vi "Periodic Tasks.vi"(0 "error in":errorcluster) -> ()   [LabVIEW 2018]
doc: "This VI runs in parallel to other tasks. It can contain as many user-defined periodic loops as you need. These can carry out PID or other sorts of timed response."
uses:
  dsinstructions.vi
  sensors.vi
  dsdata.vi
  constants.vi
  robotmodes.vi
  refnums.vi
  outputs.vi
panel:
  in  "LED Setting":dbl(slide) min=-1.0 max=1.0 step=0.01 scale=-1.0..1.0
  out "PID Tracking":cluster{"Goal Wheel Position":dbl, dbl}(graph)={"Goal Wheel Position"=0.0, -90.17571233858979}
  out "Contribution Tracking":cluster{dbl, dbl, dbl}(graph)
  in  "Swerve N-Int":i32=10 caption="N-Int"
  in  "Swerve N-Diff":i32=10 caption="N-Diff"
  in  "Swerve Kd":dbl
  in  "Swerve Ki":dbl
  in  "Swerve Kp":dbl=0.005
  out "Drive Sequencer":i32
  out "Subsystem Action":path
  out "Time Since Latch (ms)":u32
  out "Subsystem Sequencer":i32
  out "Drive Action":string
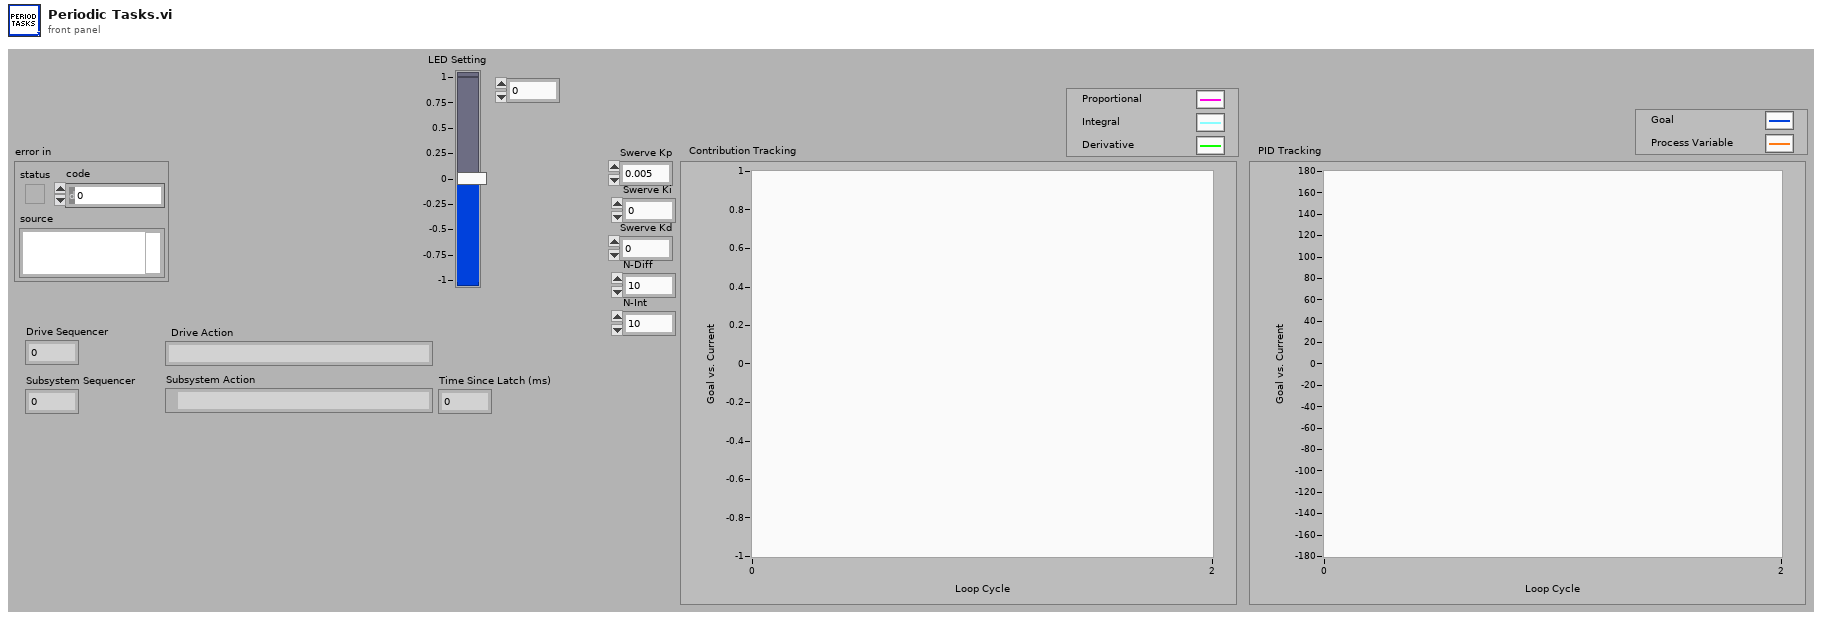
[diagram p1: front panel]
types:
  T1 = typedef "WPI_MotorControlDeviceRef.ctl" = cluster{"DeviceStatus":errorcluster, "Type":T2, "PWM":cluster{"PWM Channel":T3, "DeadBand":T4}, "CAN":cluster{"Device Number":u8, "SetOutput VI Ref":variant, "GetOutput VI Ref":variant, "Enable VI Ref":variant, "Disable VI Ref":variant, "Data":variant}, "Invert":bool, "DIO PWM":cluster{"PWM \"Enable\" Channel":T3, "DIOChannel":T5, "PWM Rate":dbl}}
  T2 = typedef "WPI_MotorControlType.ctl" = enum16{"PWM", "CAN", "DIO PWM"}
  T3 = typedef "FPGA_DIOPWMChannel.ctl" = enum8{"PWM 0", "PWM 1", "PWM 2", "PWM 3", "PWM 4", "PWM 5", "PWM 6", "PWM 7", "PWM 8", "PWM 9", "PWM MXP 0", "PWM MXP 1", "PWM MXP 2", "PWM MXP 3", "PWM MXP 4", "PWM MXP 5", "PWM MXP 6", "PWM MXP 7", "PWM MXP 8", "PWM MXP 9", "Invalid"}
  T4 = typedef "WPI_PWMDeadband.ctl" = cluster{"Name":string, "maxPositivePwm":i32, "minPositivePwm":i32, "centerPwm":i32, "maxNegativePwm":i32, "minNegativePwm":i32, "angularRange":u16}
  T5 = typedef "FPGA_DIOChannel.ctl" = enum8{"DIO 0", "DIO 1", "DIO 2", "DIO 3", "DIO 4", "DIO 5", "DIO 6", "DIO 7", "DIO 8", "DIO 9", "DIO MXP 0", "DIO MXP 1", "DIO MXP 2", "DIO MXP 3", "DIO MXP 4", "DIO MXP 5", "DIO MXP 6", "DIO MXP 7", "DIO MXP 8", "DIO MXP 9", "DIO MXP 10", "DIO MXP 11", "DIO MXP 12", "DIO MXP 13", "DIO MXP 14", "DIO MXP 15", "SPI Port CS1", "SPI Port CS2", "SPI Port CS3", "SPI Port MISO", "SPI Port MOSI", "Invalid"}
  T6 = typedef "WPI_DriverStationRobotMode2.ctl" = enum16{"Autonomous Disabled", "Autonomous Enabled", "Teleop Disabled", "Teleop Enabled", "Disconnected", "Finish", "Test Disabled", "Test Enabled", "Emergency Stopped"}
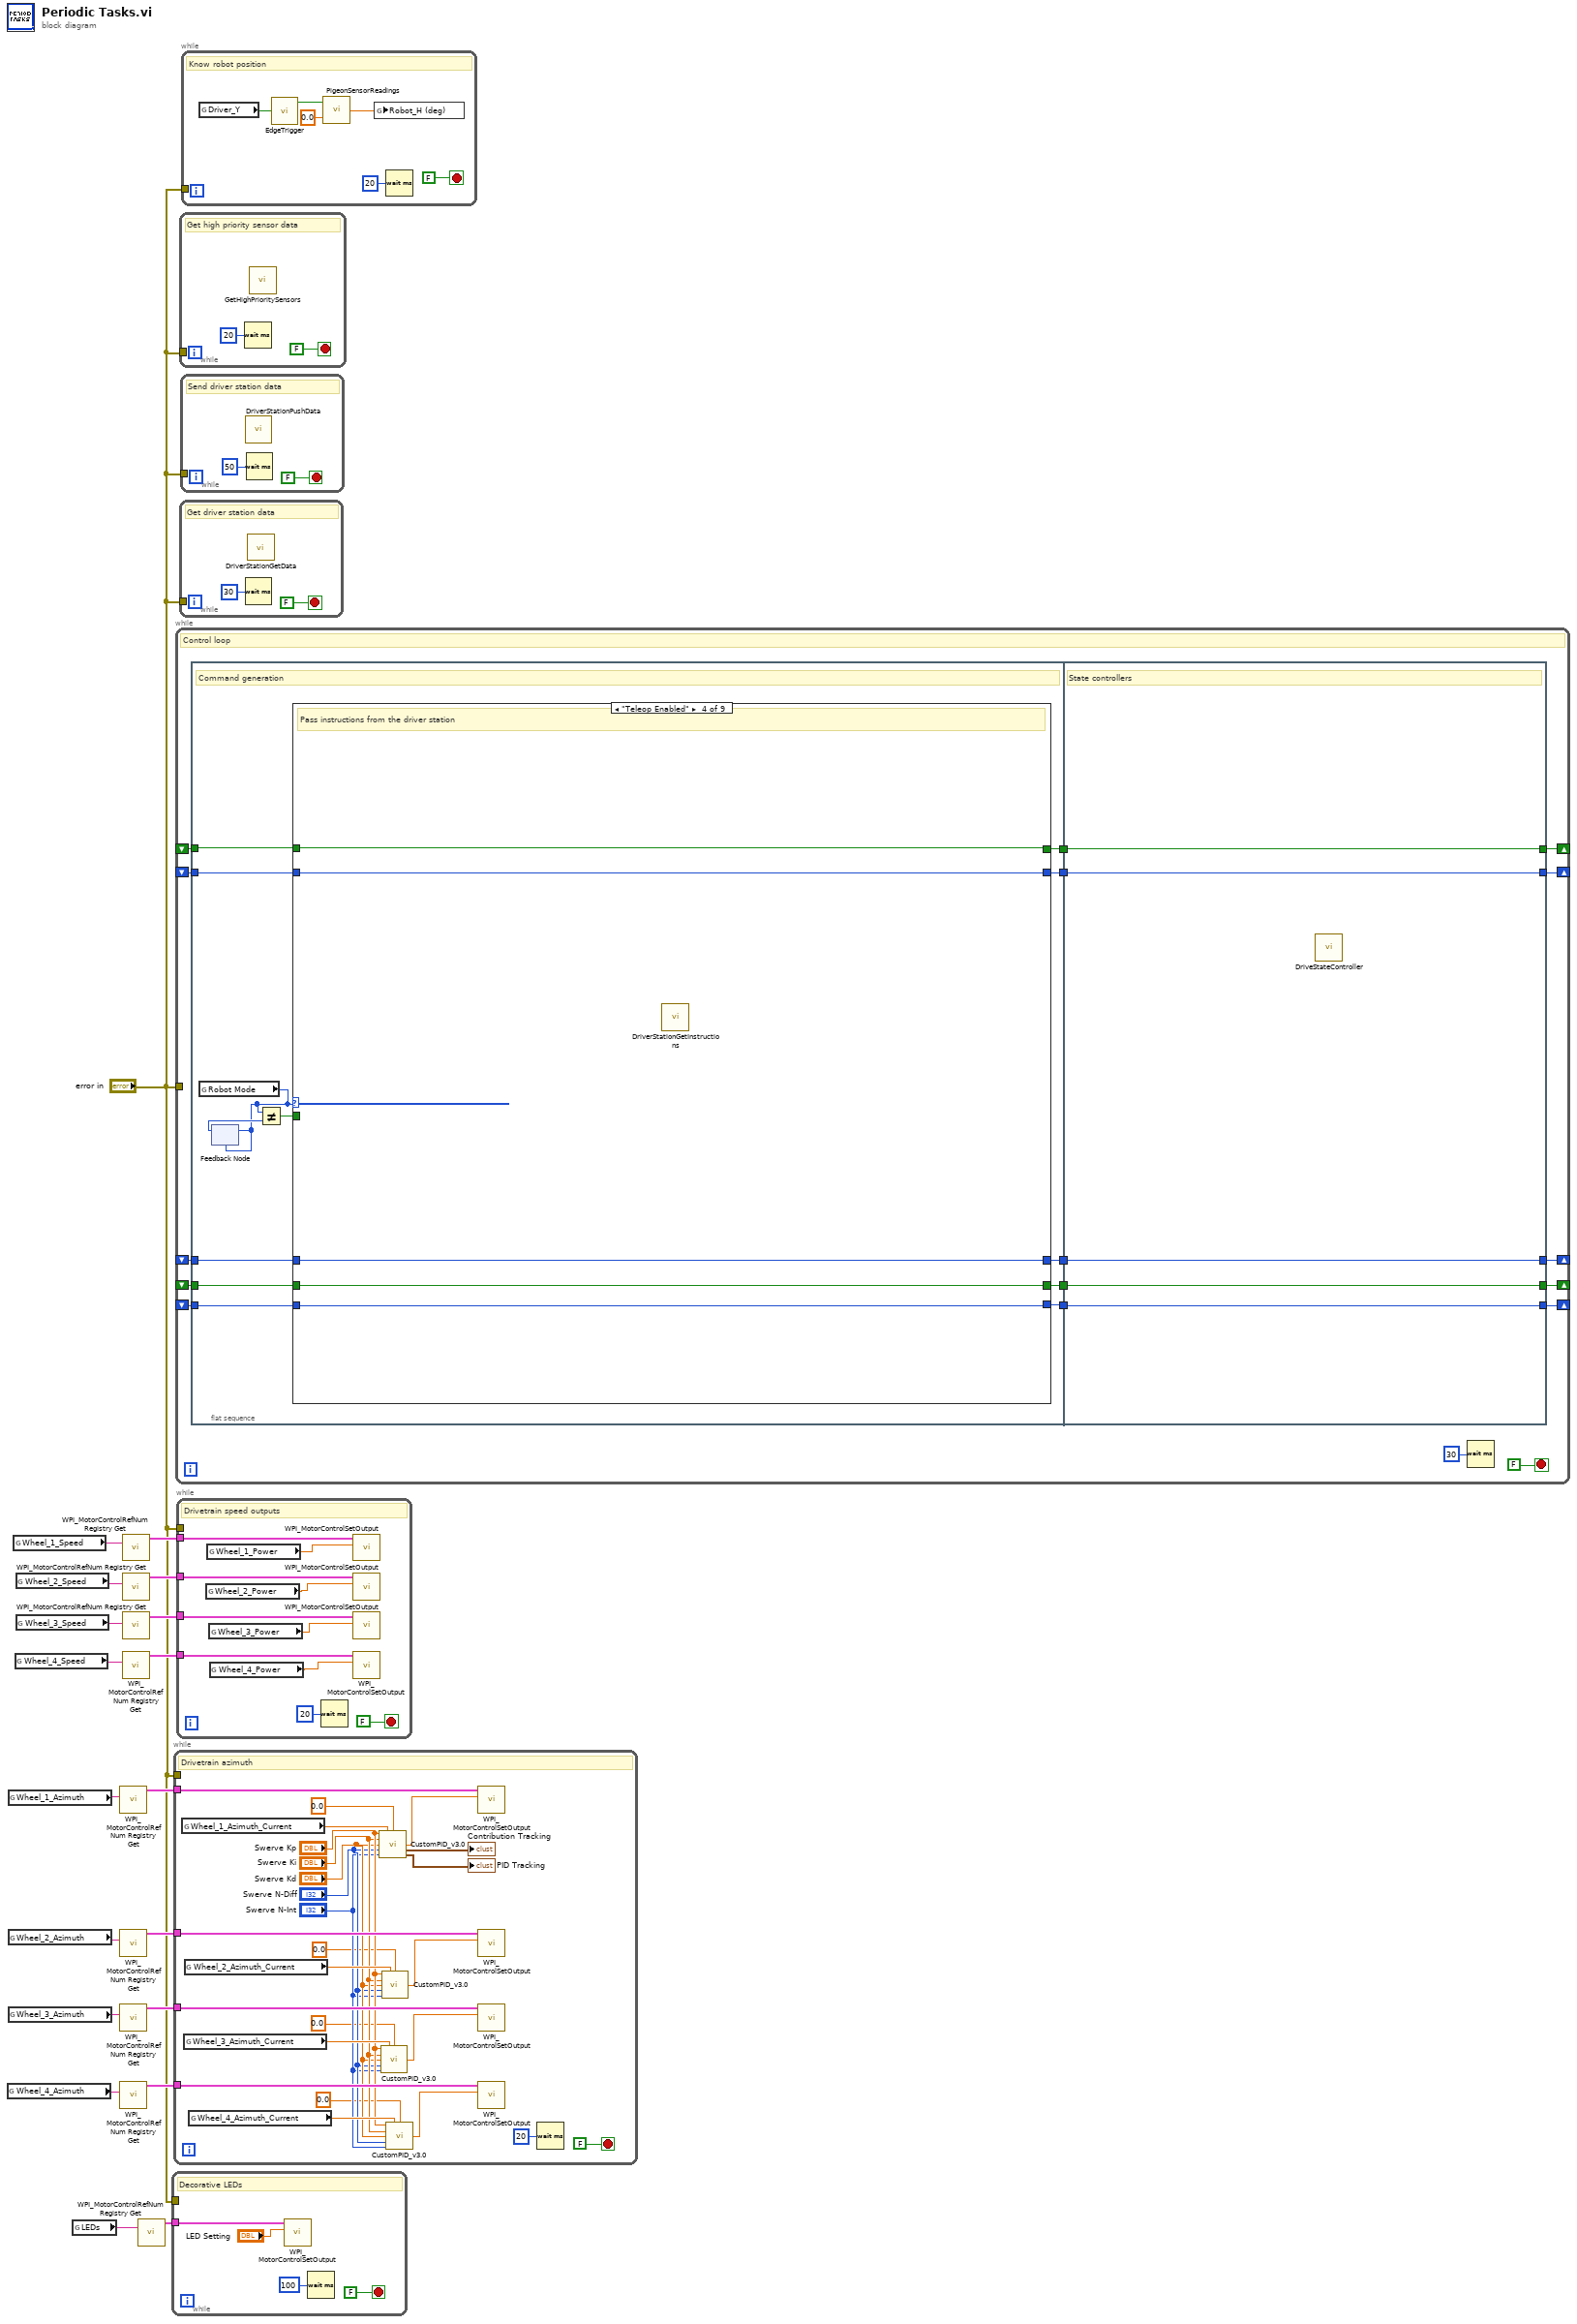
[diagram p0: block diagram]
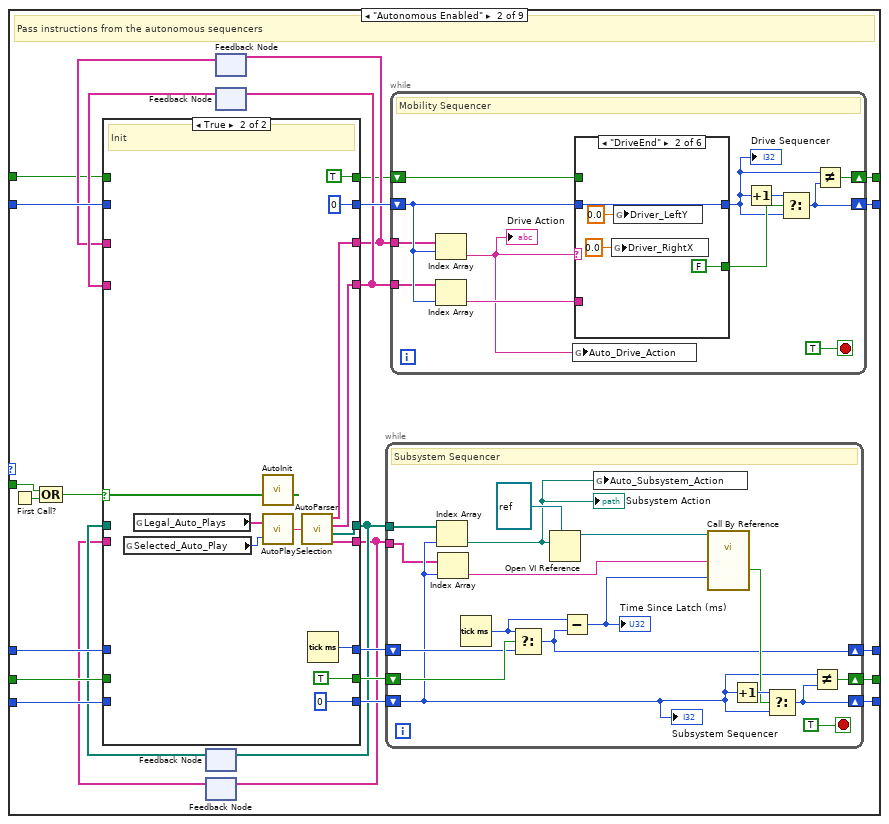
[diagram p3: hidden frame]
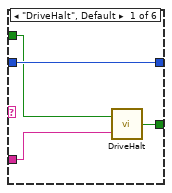
[diagram p4: hidden frame]
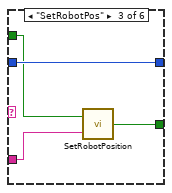
[diagram p5: hidden frame]
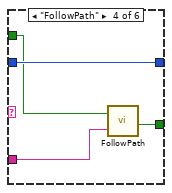
[diagram p6: hidden frame]
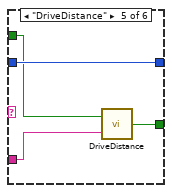
[diagram p7: hidden frame]
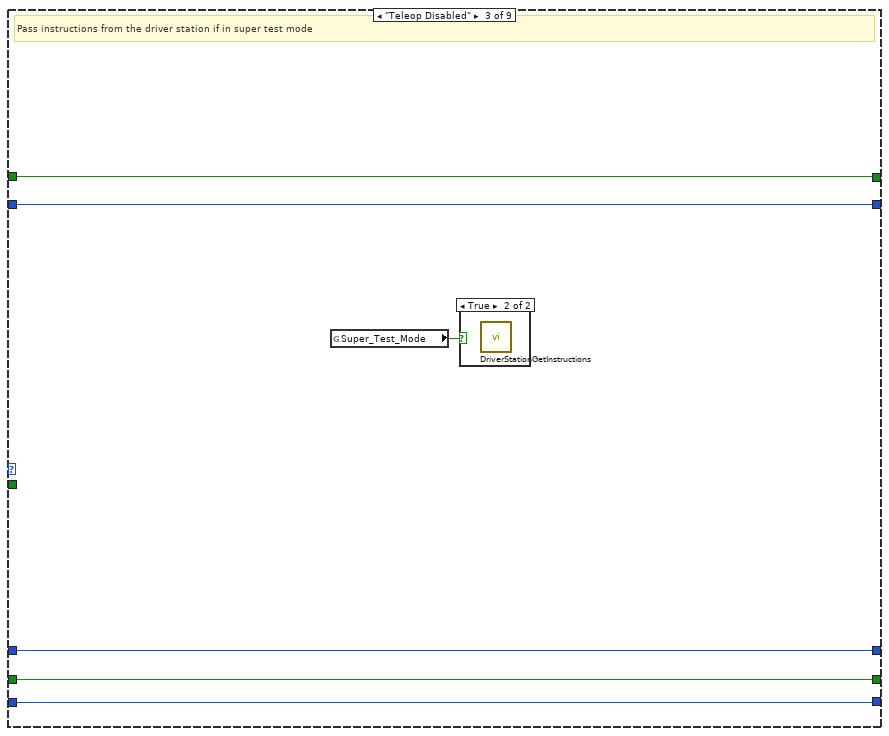
[diagram p10: hidden frame]
diagram:
  n1 = global read "refnums.vi" "Wheel_4_Azimuth"() -> (w4:string)
  n2 = global read "refnums.vi" "Wheel_1_Azimuth"() -> (w7:string)
  n3 = global read "refnums.vi" "Wheel_2_Azimuth"() -> (w6:string)
  n4 = global read "refnums.vi" "Wheel_3_Azimuth"() -> (w5:string)
  n5 = global read "refnums.vi" "Wheel_1_Speed"() -> (w15:string)
  n6 = global read "refnums.vi" "Wheel_4_Speed"() -> (w12:string)
  n7 = global read "refnums.vi" "Wheel_2_Speed"() -> (w14:string)
  n8 = global read "refnums.vi" "Wheel_3_Speed"() -> (w13:string)
  n9 = global read "refnums.vi" "LEDs"() -> (w1:string)
  n10 = call <vilib>:"WPI_MotorControlRefNum Registry Get.vi"("refnum name"=w7) -> ("MotorControlDevRef"=w11:T1)  [unwired: 9 in, 1 out]
  n11 = call <vilib>:"WPI_MotorControlRefNum Registry Get.vi"("refnum name"=w6) -> ("MotorControlDevRef"=w10:T1)  [unwired: 9 in, 1 out]
  n12 = call <vilib>:"WPI_MotorControlRefNum Registry Get.vi"("refnum name"=w5) -> ("MotorControlDevRef"=w9:T1)  [unwired: 9 in, 1 out]
  n13 = call <vilib>:"WPI_MotorControlRefNum Registry Get.vi"("refnum name"=w4) -> ("MotorControlDevRef"=w8:T1)  [unwired: 9 in, 1 out]
  n14 = call <vilib>:"WPI_MotorControlRefNum Registry Get.vi"("refnum name"=w15) -> ("MotorControlDevRef"=w19:T1)  [unwired: 9 in, 1 out]
  n15 = call <vilib>:"WPI_MotorControlRefNum Registry Get.vi"("refnum name"=w14) -> ("MotorControlDevRef"=w18:T1)  [unwired: 9 in, 1 out]
  n16 = call <vilib>:"WPI_MotorControlRefNum Registry Get.vi"("refnum name"=w13) -> ("MotorControlDevRef"=w17:T1)  [unwired: 9 in, 1 out]
  n17 = call <vilib>:"WPI_MotorControlRefNum Registry Get.vi"("refnum name"=w12) -> ("MotorControlDevRef"=w16:T1)  [unwired: 9 in, 1 out]
  n18 = call <vilib>:"WPI_MotorControlRefNum Registry Get.vi"("refnum name"=w1) -> ("MotorControlDevRef"=w2:T1)  [unwired: 9 in, 1 out]
  n19 = while {
    tunnel: "error in" -> [_]
    tunnel: w2 -> [w21]
    stop <- FALSE stop-if-true
    # "Decorative LEDs"
    n20 = call <vilib>:"WPI_MotorControlSetOutput.vi"("Output"="LED Setting", "MotorControlDevRef"=w21) -> ()  [unwired: 7 in, 3 out]
    n21 = Wait (ms)(milliseconds to wait=u32 100) -> ()  [unwired: 1 out]
  }
  n22 = while {
    tunnel: w11 -> [w46]
    tunnel: w10 -> [w45]
    tunnel: w9 -> [w44]
    tunnel: w8 -> [w43]
    tunnel: "error in" -> [_]
    stop <- FALSE stop-if-true
    # "Drivetrain azimuth"
    n23 = global read "outputs.vi" "Wheel_1_Azimuth_Current"() -> (w37:dbl)
    n24 = global read "outputs.vi" "Wheel_3_Azimuth_Current"() -> (w41:dbl)
    n25 = global read "outputs.vi" "Wheel_2_Azimuth_Current"() -> (w39:dbl)
    n26 = global read "outputs.vi" "Wheel_4_Azimuth_Current"() -> (w42:dbl)
    n27 = call "CustomPID_v3.0.vi"("Kp"="Swerve Kp", "Process Variable"=w37, "Goal"=0.0, "Ki"="Swerve Ki", "Kd"="Swerve Kd", "N-Diff"="Swerve N-Diff", "N-Int"="Swerve N-Int") -> ("Command"=w36:dbl, "Contribution Tracking"=→"Contribution Tracking":cluster{dbl, dbl, dbl}, "PID Tracking"=→"PID Tracking":cluster{"Goal Wheel Position":dbl, dbl})  [unwired: 5 in, 1 out]
    n28 = call "CustomPID_v3.0.vi"("Kp"="Swerve Kp", "Process Variable"=w41, "Goal"=0.0, "Ki"="Swerve Ki", "Kd"="Swerve Kd", "N-Diff"="Swerve N-Diff", "N-Int"="Swerve N-Int") -> ("Command"=w24:dbl)  [unwired: 5 in, 3 out]
    n29 = call "CustomPID_v3.0.vi"("Kp"="Swerve Kp", "Process Variable"=w39, "Goal"=0.0, "Ki"="Swerve Ki", "Kd"="Swerve Kd", "N-Diff"="Swerve N-Diff", "N-Int"="Swerve N-Int") -> ("Command"=w38:dbl)  [unwired: 5 in, 3 out]
    n30 = call "CustomPID_v3.0.vi"("Kp"="Swerve Kp", "Process Variable"=w42, "Goal"=0.0, "Ki"="Swerve Ki", "Kd"="Swerve Kd", "N-Diff"="Swerve N-Diff", "N-Int"="Swerve N-Int") -> ("Command"=w40:dbl)  [unwired: 5 in, 3 out]
    n31 = call <vilib>:"WPI_MotorControlSetOutput.vi"("Output"=w36, "MotorControlDevRef"=w46) -> ()  [unwired: 7 in, 3 out]
    n32 = call <vilib>:"WPI_MotorControlSetOutput.vi"("Output"=w38, "MotorControlDevRef"=w45) -> ()  [unwired: 7 in, 3 out]
    n33 = call <vilib>:"WPI_MotorControlSetOutput.vi"("Output"=w24, "MotorControlDevRef"=w44) -> ()  [unwired: 7 in, 3 out]
    n34 = call <vilib>:"WPI_MotorControlSetOutput.vi"("Output"=w40, "MotorControlDevRef"=w43) -> ()  [unwired: 7 in, 3 out]
    n35 = Wait (ms)(milliseconds to wait=u32 20) -> ()  [unwired: 1 out]
  }
  n36 = while {
    tunnel: "error in" -> [_]
    shift-right: [w55] -> _
    shift-left: _ -> [w61]
    shift-right: [w56] -> _
    shift-left: _ -> [w62]
    shift-right: [w57] -> _
    shift-left: _ -> [w63]
    shift-right: [w53] -> _
    shift-left: _ -> [w52]
    shift-right: [w50] -> _
    shift-left: _ -> [w49]
    stop <- FALSE stop-if-true
    # "Control loop"
    n37 = flat-sequence {
      tunnel: w63 -> [w75]
      tunnel: w62 -> [w74]
      tunnel: w61 -> [w73]
      tunnel: [w78] -> w60
      tunnel: [w77] -> w59
      tunnel: [w76] -> w58
      tunnel: [w70] -> w54
      tunnel: w52 -> [w69]
      tunnel: [w68] -> w51
      tunnel: w49 -> [w67]
      tunnel: w60 -> [w221]
      tunnel: w59 -> [w220]
      tunnel: w58 -> [w219]
      tunnel: [w221] -> w57
      tunnel: [w220] -> w56
      tunnel: [w219] -> w55
      tunnel: w54 -> [w218]
      tunnel: [w218] -> w53
      tunnel: [w217] -> w50
      tunnel: w51 -> [w217]
      frame #0 {
        # "Command generation"
        n38 = global read "dsdata.vi" "Robot Mode"() -> (w66:T6)
        n39 = feedback-in #1(w66) -> ()
        n40 = feedback #1(w66) -> (w72:T6)
        n41 = Not Equal?(x=w66, y=w72) -> (x != y?=w71:bool)
        n42 = case shown="\"Teleop Enabled\"" w66 {
          tunnel: w75 -> [w83 w106 w184 w189 w194 w199 w204 w209 w214]
          tunnel: w74 -> [w82 w104 w183 w188 w193 w198 w203 w208 w213]
          tunnel: w73 -> [w81 w103 w182 w187 w192 w197 w202 w207 w212]
          tunnel: [w83 w109 w184 w189 w194 w199 w204 w209 w214] -> w78
          tunnel: [w82 w108 w183 w188 w193 w198 w203 w208 w213] -> w77
          tunnel: [w81 w107 w182 w187 w192 w197 w202 w207 w212] -> w76
          tunnel: w71 -> [_ w98 _ _ _ _ _ _ _]
          tunnel: [w80 w92 w185 w190 w195 w200 w205 w210 w215] -> w70
          tunnel: w69 -> [w80 w91 w185 w190 w195 w200 w205 w210 w215]
          tunnel: [w79 w85 w186 w191 w196 w201 w206 w211 w216] -> w68
          tunnel: w67 -> [w79 w84 w186 w191 w196 w201 w206 w211 w216]
          frame "Autonomous Disabled", Default {
          }
          frame "Autonomous Enabled" {
            # "Pass instructions from the autonomous sequencers"
            n43 = First Call?() -> (First Call?: T/F=w99:bool)
            n44 = Compound Arithmetic op=OR(w98, w99) -> (w100:bool)
            n45 = feedback #2() -> (w95:path[])  [unwired: 1 in]
            n46 = feedback #3() -> (w94:string[])  [unwired: 1 in]
            n47 = feedback #4() -> (w87:string[])  [unwired: 1 in]
            n48 = feedback #5() -> (w88:string[])  [unwired: 1 in]
            n49 = case shown="True" w100 {
              tunnel: w103 -> [w149 _]
              tunnel: w104 -> [w150 _]
              tunnel: w106 -> [w151 _]
              tunnel: [w151 w163] -> w105
              tunnel: [w150 TRUE ("Advance Trigger")] -> w102
              tunnel: [w149 0] -> w101
              tunnel: [w148 w156] -> w97
              tunnel: [w147 w160] -> w96
              tunnel: w95 -> [w148 _]
              tunnel: w94 -> [w147 _]
              tunnel: [w146 0] -> w93
              tunnel: w91 -> [w146 _]
              tunnel: [w145 w158] -> w90
              tunnel: [w144 w157] -> w89
              tunnel: w88 -> [w145 _]
              tunnel: w87 -> [w144 _]
              tunnel: [w143 TRUE] -> w86
              tunnel: w84 -> [w143 _]
              frame False {
                # "Pass"
              }
              frame True {
                # "Init"
                n50 = global read "dsdata.vi" "Selected_Auto_Play"() -> (w154:u16)
                n51 = global read "constants.vi" "Legal_Auto_Plays"() -> (w153:string[])
                n52 = call "AutoInit.vi"() -> ()  [unwired: 1 in]
                n53 = call "AutoPlaySelection.vi"("Selected Auto Play"=w154, "Auto Plays"=w153) -> ("Autonomous Commands"=w152:string)
                n54 = call "AutoParser.vi"("Auto Play"=w152) -> ("Drive Mode Strings"=w157:string[], "Drive Command Strings"=w158:string[], "Subsystem VI References"=w156:path[], "Subsystem Command Strings"=w160:string[])
                n55 = Tick Count (ms)() -> (millisecond timer value=w163:u32)
              }
            }
            n56 = feedback-in #2(w97) -> ()
            n57 = feedback-in #3(w96) -> ()
            n58 = feedback-in #4(w89) -> ()
            n59 = feedback-in #5(w90) -> ()
            n60 = while {
              tunnel: w97 -> [w168]
              shift-right: [w176] -> w107
              shift-left: w101 -> [w167]
              shift-right: [w175] -> w108
              shift-left: w102 -> [w174]
              shift-right: [w172] -> w109
              shift-left: w105 -> [w173]
              tunnel: w96 -> [w166]
              stop <- TRUE stop-if-true
              # "Subsystem Sequencer"
              n61 = Index Array(array=w168, index=w167) -> (element=w164:path)
              "Subsystem Action" <- w164
              n62 = Index Array(array=w166, index=w167) -> (element=w165:string)
              n63 = Tick Count (ms)() -> (millisecond timer value=w171:u32)
              n64 = Select(t=w171, s=w174, f=w173) -> (s? t:f=w172:u32)
              n65 = Open VI Reference(type specifier VI Refnum (for type only)=refnum<vi> refnum, vi path=w164) -> (vi reference=w170:refnum<vi>)  [unwired: 4 in, 1 out]
              n66 = Subtract(x=w171, y=w172) -> (x-y=w169:u32)
              "Time Since Latch (ms)" <- w169
              n67 = global write "robotmodes.vi" "Auto_Subsystem_Action"(w164) -> ()
              n68 = call-by-ref "?"(reference=w170, "Time Since Latch"=w169, "Instruction String"=w165) -> ("Advance Trigger"=w177:bool)  [unwired: 1 in, 2 out]
              n69 = Increment(x=w167) -> (x+1=w179:i32)
              n70 = Select(t=w179, s=w177, f=w167) -> (s? t:f=w176:i32)
              n71 = Not Equal?(x=w167, y=w176) -> (x != y?=w175:bool)
              "Subsystem Sequencer" <- w167
            }
            n72 = while {
              shift-right: [w114] -> w92
              shift-left: w93 -> [w119]
              tunnel: w89 -> [w118]
              tunnel: w90 -> [w117]
              shift-right: [w113] -> w85
              shift-left: w86 -> [w112]
              stop <- TRUE stop-if-true
              # "Mobility Sequencer"
              n73 = Index Array(array=w118, index=w119) -> (element=w110:string)
              "Drive Action" <- w110
              n74 = Index Array(array=w117, index=w119) -> (element=w116:string)
              n75 = global write "robotmodes.vi" "Auto_Drive_Action"(w110) -> ()
              n76 = case shown="\"DriveEnd\"" w110 {
                tunnel: w119 -> [w125 w129 w133 w137 w141 w142]
                tunnel: [w125 w129 w133 w137 w141 w142] -> w111
                tunnel: w116 -> [w122 _ w131 w134 w139 _]
                tunnel: [w124 FALSE ("Increment") w132 w136 w138 _] -> w115
                tunnel: w112 -> [w123 _ w130 w135 w140 _]
                frame "DriveHalt", Default {
                  n77 = call "DriveHalt.vi"("Parameter String"=w122, "Reinit"=w123) -> ("Increment"=w124:bool)
                }
                frame "DriveEnd" {
                  n78 = global write "dsinstructions.vi" "Driver_RightX"(0.0 ("Driver_RightX")) -> ()
                  n79 = global write "dsinstructions.vi" "Driver_LeftY"(0.0 ("Driver_LeftY")) -> ()
                }
                frame "SetRobotPos" {
                  n80 = call "SetRobotPosition.vi"("Parameter String"=w131, "Reinit"=w130) -> ("Increment"=w132:bool)
                }
                frame "FollowPath" {
                  n81 = call "FollowPath.vi"("Parameter String"=w134, "Reinit"=w135) -> ("Increment"=w136:bool)
                }
                frame "DriveDistance" {
                  n82 = call "DriveDistance.vi"("Parameter String"=w139, "Reinit"=w140) -> ("Increment"=w138:bool)
                }
                frame "RotateAngle" {
                }
              }
              "Drive Sequencer" <- w111
              n83 = Increment(x=w111) -> (x+1=w120:i32)
              n84 = Select(t=w120, s=w115, f=w111) -> (s? t:f=w114:i32)
              n85 = Not Equal?(x=w111, y=w114) -> (x != y?=w113:bool)
            }
          }
          frame "Teleop Disabled" {
            # "Pass instructions from the driver station if in super test mode"
            n86 = global read "dsdata.vi" "Super_Test_Mode"() -> (w181:bool)
            n87 = case shown="True" w181 {
              frame False {
              }
              frame True {
                n88 = call "DriverStationGetInstructions.vi"() -> ()  [unwired: 12 in]
              }
            }
          }
          frame "Teleop Enabled" {
            # "Pass instructions from the driver station"
            n89 = call "DriverStationGetInstructions.vi"() -> ()  [unwired: 12 in]
          }
          frame "Finish" {
            # "Clean up operations are in the Finish.vi in RobotMain.vi"
          }
          frame "Test Disabled" {
            # "We are not using the testing mode"
          }
          frame "Test Enabled" {
            # "We are not using the testing mode"
          }
          frame "Disconnected" {
          }
          frame "Emergency Stopped" {
          }
        }
      }
      frame #1 {
        # "State controllers"
        n90 = call "DriveStateController.vi"() -> ()  [unwired: 1 in]
      }
    }
    n91 = Wait (ms)(milliseconds to wait=u32 30) -> ()  [unwired: 1 out]
  }
  n92 = while {
    tunnel: "error in" -> [_]
    tunnel: w19 -> [w229]
    tunnel: w18 -> [w228]
    tunnel: w17 -> [w227]
    tunnel: w16 -> [w226]
    stop <- FALSE stop-if-true
    # "Drivetrain speed outputs"
    n93 = global read "outputs.vi" "Wheel_2_Power"() -> (w224:dbl)
    n94 = global read "outputs.vi" "Wheel_1_Power"() -> (w225:dbl)
    n95 = global read "outputs.vi" "Wheel_3_Power"() -> (w222:dbl)
    n96 = global read "outputs.vi" "Wheel_4_Power"() -> (w223:dbl)
    n97 = Wait (ms)(milliseconds to wait=u32 20) -> ()  [unwired: 1 out]
    n98 = call <vilib>:"WPI_MotorControlSetOutput.vi"("Output"=w225, "MotorControlDevRef"=w229) -> ()  [unwired: 7 in, 3 out]
    n99 = call <vilib>:"WPI_MotorControlSetOutput.vi"("Output"=w224, "MotorControlDevRef"=w228) -> ()  [unwired: 7 in, 3 out]
    n100 = call <vilib>:"WPI_MotorControlSetOutput.vi"("Output"=w222, "MotorControlDevRef"=w227) -> ()  [unwired: 7 in, 3 out]
    n101 = call <vilib>:"WPI_MotorControlSetOutput.vi"("Output"=w223, "MotorControlDevRef"=w226) -> ()  [unwired: 7 in, 3 out]
  }
  n102 = while {
    tunnel: "error in" -> [_]
    stop <- FALSE stop-if-true
    # "Get high priority sensor data"
    n103 = Wait (ms)(milliseconds to wait=u32 20) -> ()  [unwired: 1 out]
    n104 = call "GetHighPrioritySensors.vi"() -> ()  [unwired: 1 in]
  }
  n105 = while {
    tunnel: "error in" -> [_]
    stop <- FALSE stop-if-true
    # "Get driver station data"
    n106 = Wait (ms)(milliseconds to wait=u32 30) -> ()  [unwired: 1 out]
    n107 = call "DriverStationGetData.vi"() -> ()  [unwired: 1 in]
  }
  n108 = while {
    tunnel: "error in" -> [_]
    stop <- FALSE stop-if-true
    # "Send driver station data"
    n109 = call "DriverStationPushData.vi"() -> ()  [unwired: 12 in]
    n110 = Wait (ms)(milliseconds to wait=u32 50) -> ()  [unwired: 1 out]
  }
  n111 = while {
    tunnel: "error in" -> [_]
    stop <- FALSE stop-if-true
    # "Know robot position"
    n112 = global read "dsinstructions.vi" "Driver_Y"() -> (w240:bool)
    n113 = call "EdgeTrigger.vi"("Input Signal"=w240) -> ("Rising Edge Trigger"=w241:bool)  [unwired: 2 out]
    n114 = call "PigeonSensorReadings.vi"("Reset Yaw (deg)"=0.0, "Reset Yaw"=w241) -> ("Yaw (deg)"=w239:dbl)
    n115 = global write "sensors.vi" "Robot_H (deg)"(w239) -> ()
    n116 = Wait (ms)(milliseconds to wait=u32 20) -> ()  [unwired: 1 out]
  }
